vi "USBTC08GetSingle.vi"(6 "Units":enum16{"C°", "F°", "K°", "R°"}(ring), 8 "error in (no error)":errorcluster, 11 "Handle in":i16) -> (0 "error out":errorcluster, 1 "Overflow":i16, 2 "Array out":sgl[](array[numeric]), 3 "Handle out":i16)   [LabVIEW 2010]
uses:
  usbtc08.dll
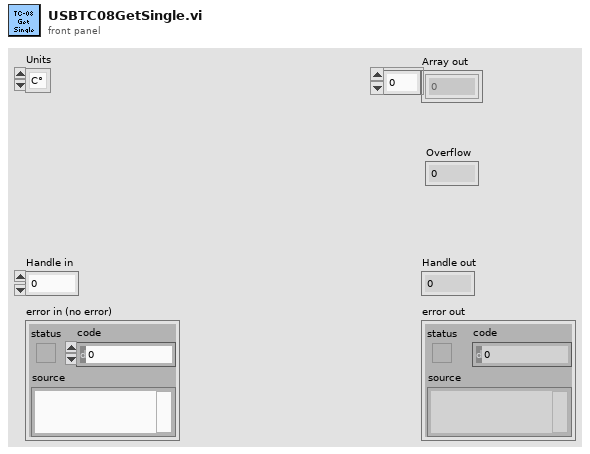
[diagram p1: front panel]
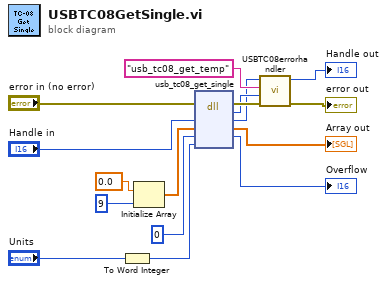
[diagram p0: block diagram]
diagram:
  n1 = To Word Integer(number="Units") -> (16bit integer=w2:i16)
  n2 = Initialize Array(sgl 0.0, i16 9) -> (w9:sgl[])
  n3 = dll-call lib="usbtc08.dll" fn="usb_tc08_get_single"(error in="error in (no error)", "handle"="Handle in", "temp_buffer"=w9, "overflow"=i16 0, "units"=w2) -> (error out=w12:errorcluster, "return type"=w4:i16, "handle"=w3:i16, "temp_buffer"=→"Array out":sgl[], "overflow"=→"Overflow":i16)  [unwired: 3 in, 1 out]
  n4 = call "USBTC08errorhandler.vi"("error in (no error)"=w12, "Return"=w4, "API function"="usb_tc08_get_temp", "Handle in"=w3) -> ("error out"=→"error out":errorcluster, "Handle out"=→"Handle out":i16)  [unwired: 6 in]
